vi "Arm Feed Forward.vi"(10 "Numeric":i32, 11 "Arm Position":dbl) -> (3 "Feed Forward":dbl)   [LabVIEW 2014]
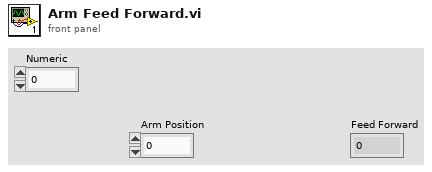
[diagram p1: front panel]
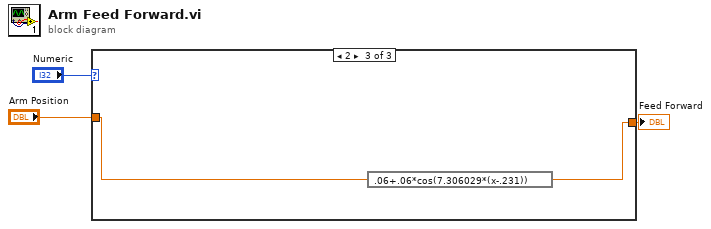
[diagram p0: block diagram]
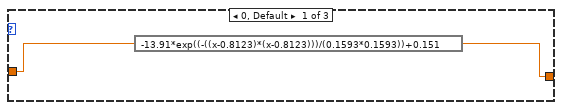
[diagram p2: hidden frame]
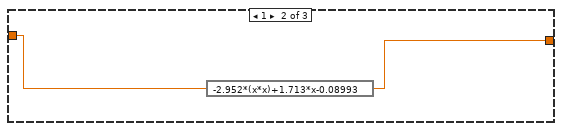
[diagram p3: hidden frame]
diagram:
  n1 = case shown="2" "Numeric" {
    tunnel: "Arm Position" -> [w5 w7 w8]
    tunnel: [w4 w6 w9] -> w2
    frame 0, Default {
      n2 = expression code="-13.91*exp((-((x-0.8123)*(x-0.8123)))/(0.1593*0.1593))+0.151"(w5) -> (w4:dbl)
    }
    frame 1 {
      n3 = expression code="-2.952*(x*x)+1.713*x-0.08993"(w7) -> (w6:dbl)
    }
    frame 2 {
      n4 = expression code=".06+.06*cos(7.306029*(x-.231))"(w8) -> (w9:dbl)
    }
  }
  "Feed Forward" <- w2
